vi "Dispatch Start.vi"(8 "error in (no error)":errorcluster, 11 "Dispatcher in":refnum<class "Dispatcher Thread.lvclass">) -> (0 "error out":errorcluster, 3 "Dispatcher out":refnum<class "Dispatcher Thread.lvclass">)   [LabVIEW 2021, in "DSF Core.lvlib" / "Dispatcher Thread.lvclass"]
uses:
  Dispatcher Thread.lvclass
  Dispatcher Thread.lvclass/Dispatcher Thread.ctl
  Interface/Dispatcher/Response.ctl
  Interface/Dispatcher/Response Data.ctl
  Interface/Dispatcher/Parameters.ctl
  Interface/Dispatcher/Dispatcher Interface.lvclass
  Interface/Plugin/Plugin Interface.lvclass
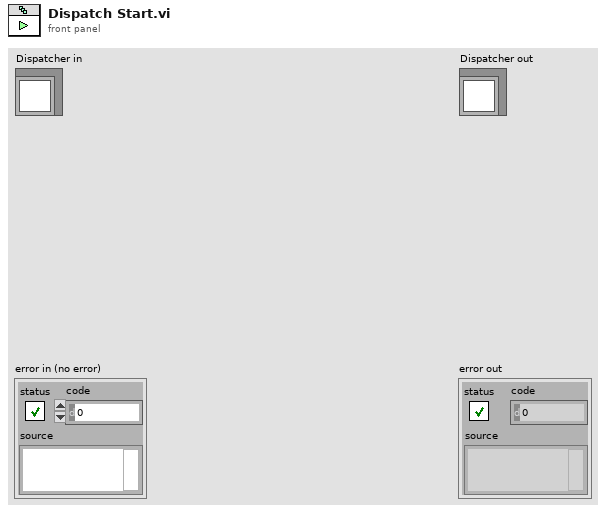
[diagram p1: front panel]
types:
  T1 = typedef "DSF Core.lvlib/Dispatcher Interface.lvclass/Response.ctl" = enum8{"General Ack", "Error", "Shutting Down"}
  T2 = typedef "DSF Core.lvlib/Dispatcher Interface.lvclass/Response Data.ctl" = cluster{"Response":T1, "Parameters":T3}
  T3 = typedef "DSF Core.lvlib/Dispatcher Interface.lvclass/Parameters.ctl" = cluster{"arg1":u64, "arg2":u64}
  T4 = typedef "DSF Core.lvlib/Dispatcher Thread.lvclass/Plugin Settings.ctl" = cluster{"Transfer Group threads":i32[], "Plugin Thread Interfaces":refnum<class "Plugin Interface.lvclass">[]}
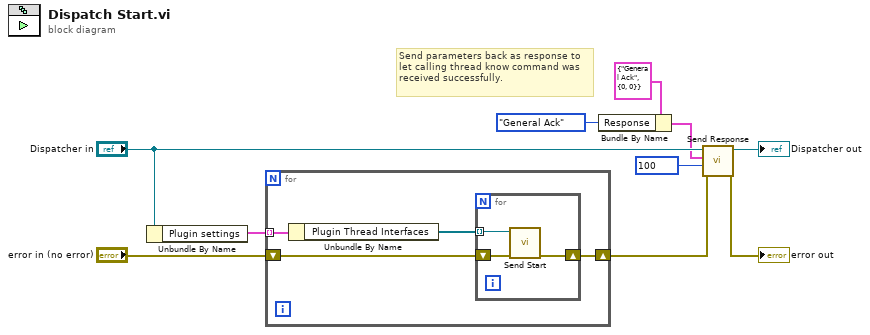
[diagram p0: block diagram]
diagram:
  # "Send parameters back as response to let calling thread know command was received successfully."
  n1 = Unbundle By Name("Dispatcher in") -> ("Plugin settings"=w10:T4[])
  n2 = for {
    tunnel: w10 -> [w12] mode=indexing
    shift-right: [w14] -> w7
    shift-left: "error in (no error)" -> [w13]
    n3 = Unbundle By Name(w12) -> ("Plugin Thread Interfaces"=w11:refnum<class "Plugin Interface.lvclass">[])
    n4 = for {
      tunnel: w11 -> [w17] mode=indexing
      shift-right: [w15] -> w14
      shift-left: w13 -> [w16]
      n5 = call "Send Start.vi"("error in (no error)"=w16, "Plugin Interface in"=w17) -> ("error out"=w15:errorcluster)  [unwired: 8 in, 1 out]
    }
  }
  n6 = Bundle By Name(cluster=T2 {"Response"=enum."General Ack", "Parameters"={"arg1"=0, "arg2"=0}} ("response"), "Response"=Response."General Ack") -> (w1:T2)
  n7 = call "Send Response.vi"("error in (no error)"=w7, "timeout in ms (0)"=100, "response"=w1, "Dispatcher in"="Dispatcher in") -> ("error out"=→"error out":errorcluster, "Dispatcher out"=→"Dispatcher out":refnum<class "Dispatcher Thread.lvclass">)  [unwired: 6 in]
